vi "Get Arguments.vi"(8 "error in (no error)":errorcluster caption="entrée d'erreur (pas d'erreur)", 11 "Class Instrument Process en entrée":refnum<class "Class Instrument Process.lvclass">) -> (0 "error out":errorcluster caption="sortie d'erreur", 2 "Arguments":string, 3 "Class Instrument Process en sortie":refnum<class "Class Instrument Process.lvclass">)   [LabVIEW 2020, in "Library Instrument & Equipement.lvlib" / "Library Instruments.lvlib" / "Class Instrument Process.lvclass"]
uses:
  Class Instrument Process.lvclass
  Class Instrument Process.lvclass/Class Instrument Process.ctl
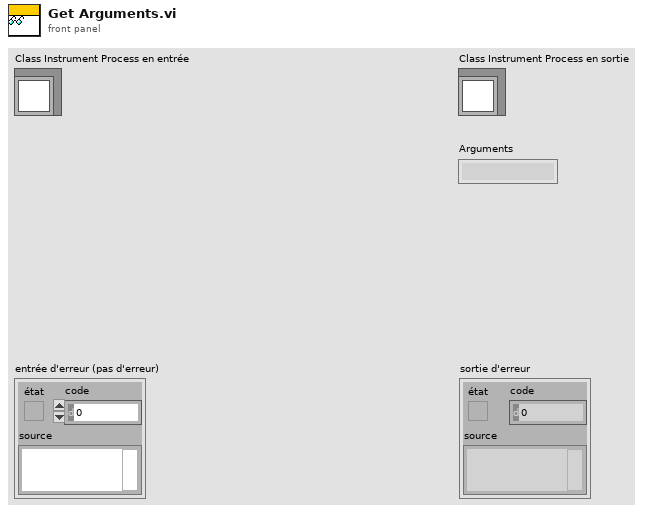
[diagram p1: front panel]
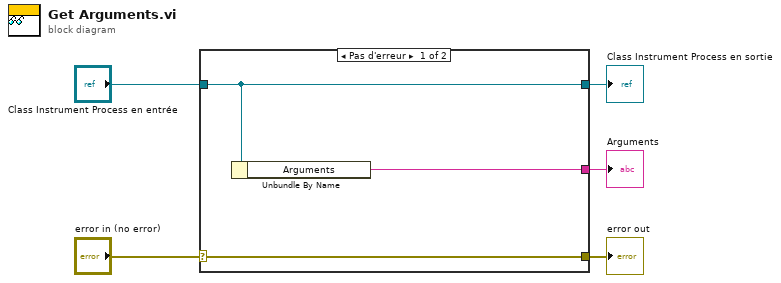
[diagram p0: block diagram]
diagram:
  n1 = case shown="Pas d'erreur" "error in (no error)" {
    selector: "error in (no error)" -> [w8 w9]
    tunnel: [w8 w9] -> w4
    tunnel: [w7 w10] -> w2
    tunnel: "Class Instrument Process en entrée" -> [w7 w10]
    tunnel: [w6 _] -> w1
    frame No Error {
      n2 = Unbundle By Name(w7) -> ("Arguments"=w6:string)
    }
    frame Error {
    }
  }
  "error out" <- w4
  "Class Instrument Process en sortie" <- w2
  "Arguments" <- w1
